vi "I2C Indexer(David Documentation).vi"(10 "Decrement?":bool, 11 "Load?":bool) -> (3 "Numeric":fxp<+,3,3>)   [LabVIEW 2015]
doc: "This VI configures the counting down."
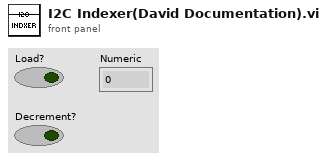
[diagram p1: front panel]
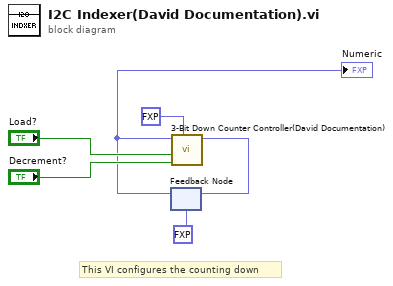
[diagram p0: block diagram]
diagram:
  # "This VI configures the counting down"
  n1 = feedback #1(fxp<+,3,3> 0.0) -> (w3:fxp<+,3,3>)
  "Numeric" <- w3
  n2 = call "3-Bit Down Counter Controller(David Documentation).vi"("Input"=fxp<+,3,3> 7.0 ("Value"), "Decrement?"="Decrement?", "Load?"="Load?", "Value"=w3) -> ("Value+"=w2:fxp<+,3,3>)  [unwired: 7 in]
  n3 = feedback-in #1(w2) -> ()
